vi "NewList.vi"(8 "error in (no error)":errorcluster, 9 "Titles":string[](array[string]), 10 "Contents":string[][](array[string]), 11 "List In":refnum<class "List.lvclass">) -> (0 "error out":errorcluster, 3 "List out":refnum<class "List.lvclass">)   [LabVIEW 2015, in "List.lvclass"]
uses:
  List.lvclass
  List.lvclass/List.ctl
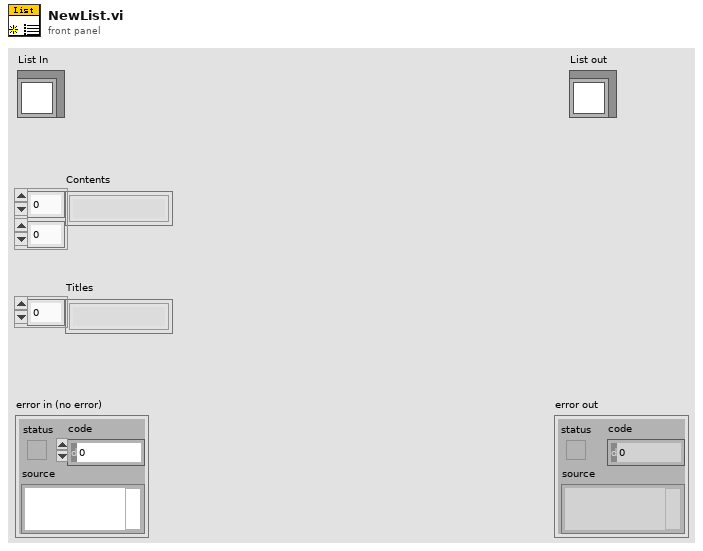
[diagram p1: front panel]
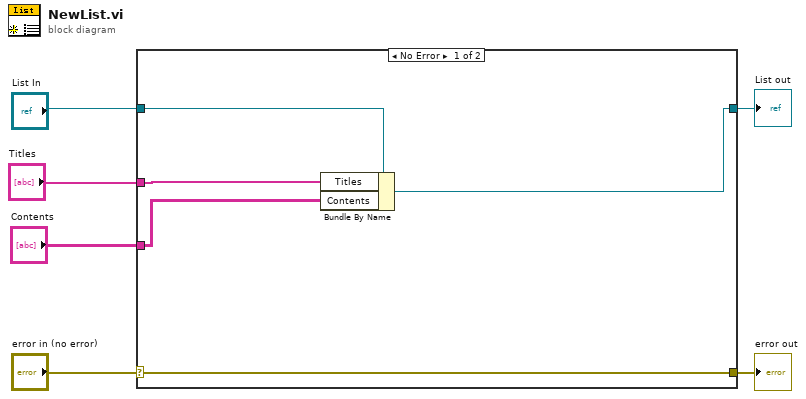
[diagram p0: block diagram]
diagram:
  n1 = case shown="No Error" "error in (no error)" {
    selector: "error in (no error)" -> [w11 w13]
    tunnel: [w11 w13] -> w5
    tunnel: [w7 w12] -> w4
    tunnel: "List In" -> [w10 w12]
    tunnel: "Contents" -> [w8 _]
    tunnel: "Titles" -> [w9 _]
    frame No Error {
      n2 = Bundle By Name(cluster=w10, "Titles"=w9, "Contents"=w8) -> (w7:refnum<class "List.lvclass">)
    }
    frame Error {
    }
  }
  "error out" <- w5
  "List out" <- w4
